vi "HeadAcousticHDF_Create.vi"(0 "reference in":refnum<class "HeadAcousticHDF.lvclass">, 5 "error in (no error)":errorcluster, 6 "Time Data":refnum<class "GSwFormDSP.lvclass">, 7 "Application Name":string, 9 "State Queue":string[](array[string])) -> (14 "reference out":refnum<class "HeadAcousticHDF.lvclass">, 19 "error out":errorcluster)   [LabVIEW 2022 SP3, in "HeadAcousticHDF.lvclass"]
doc: "Constructor."
uses:
  HeadAcousticHDF.lvclass
  C:/Program Files/National Instruments/LabVIEW 2022/vi.lib/addons/_AddQ/G#Object/G#Object.lvclass
  W:/projects/archives/23 Charette AI Group/SPWB/API/Generic Utilities_class/Generic Utilities.lvclass
  API/GSwFormDSP_class/GSwFormDSP.lvclass
  <vilib>/addons/_AddQ/G#Object/G#Object.lvclass
  API/Generic Utilities_class/Generic Utilities.lvclass
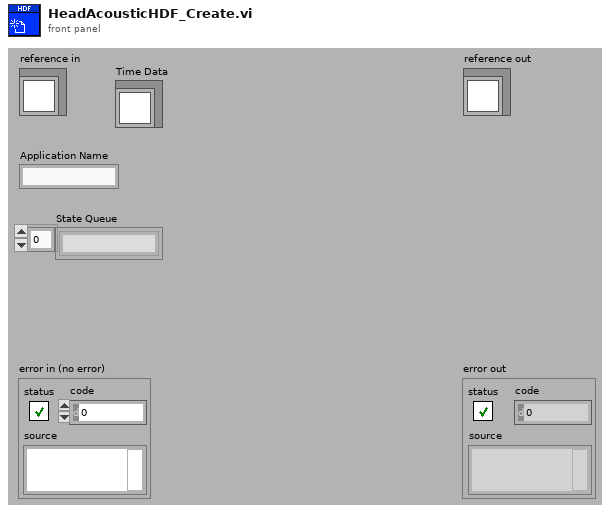
[diagram p1: front panel]
types:
  T1 = typedef "HeadAcousticHDF.lvclass/ObjectAttributesRef.ctl" = refnum<data-value>
  T2 = typedef "HeadAcousticHDF.lvclass/ObjectAttributes.ctl" = cluster{"Time Data":refnum<class "GSwFormDSP.lvclass">, "Data Plugin Name":string, "Additional Data Plugin Name":string, "New Time Data Obj?":bool}
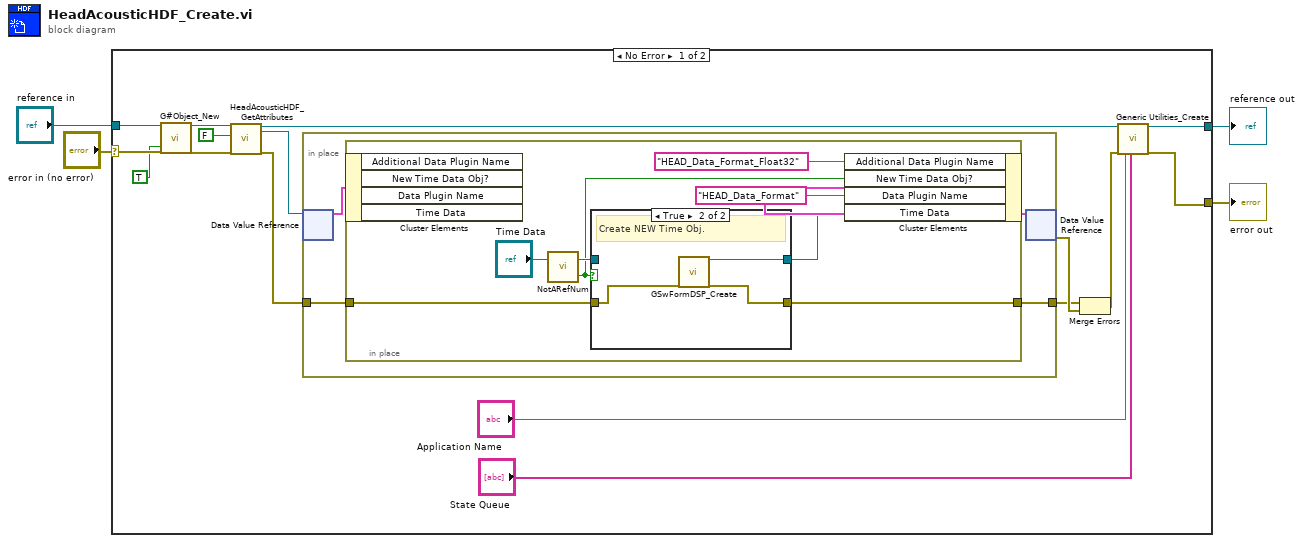
[diagram p0: block diagram]
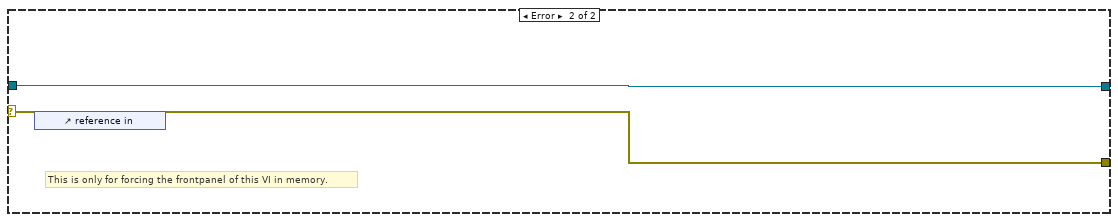
[diagram p3: hidden frame]
diagram:
  n1 = case shown="No Error" "error in (no error)" {
    selector: "error in (no error)" -> [w19 w39]
    tunnel: [w9 w39] -> w3
    tunnel: [w11 w38] -> w1
    tunnel: "reference in" -> [w20 w38]
    frame No Error {
      n2 = call <vilib>:"G#Object_New.vi"("reference in"=w20, "error in (no error)"=w19, "user counter (T)?"=TRUE ("User Counter")) -> ("reference out"=w14:refnum<class "HeadAcousticHDF.lvclass">, "error out"=w13:errorcluster)  [unwired: 14 in, 1 out]
      n3 = call "HeadAcousticHDF_GetAttributes.vi"("reference in"=w14, "return data? (T)"=FALSE ("return data"), "error in (no error)"=w13) -> ("reference out"=w12:refnum<class "HeadAcousticHDF.lvclass">, "attributes ref"=w16:T1, "error out"=w7:errorcluster)  [unwired: 13 in, 1 out]
      n4 = in-place {
        in-place-border: w7 -> [w22]
        in-place-border: [w21] -> w6
        n5 = in-place-dvr #1(w16) -> (w23:T2)  [unwired: 1 out]
        n6 = in-place {
          in-place-border: w22 -> [w30]
          in-place-border: [w29] -> w21
          n7 = in-place-cluster #2(w23) -> ()  [unwired: 4 out]
          n8 = call-dynamic "NotARefNum.vi"("reference in"="Time Data") -> ("not a refnum?"=w27:bool, "reference out"=w32:refnum<class "GSwFormDSP.lvclass">)  [unwired: 1 in]
          n9 = case shown="True" w27 {
            tunnel: [w34 w37] -> w25
            tunnel: w32 -> [w34 _]
            tunnel: w30 -> [w33 w36]
            tunnel: [w33 w35] -> w29
            frame False {
              # "Copy an existing reference."
            }
            frame True {
              # "Create NEW Time Obj."
              n10 = call "GSwFormDSP_Create.vi"("error in (no error)"=w36) -> ("reference out"=w37:refnum<class "GSwFormDSP.lvclass">, "error out"=w35:errorcluster)  [unwired: 17 in]
            }
          }
          n11 = in-place-cluster #2("Additional Data Plugin Name"="HEAD_Data_Format_Float32" ("Data Plugin Name"), "New Time Data Obj?"=w27, "Data Plugin Name"="HEAD_Data_Format", "Time Data"=w25) -> (w24:T2)
        }
        n12 = in-place-dvr #1(w24) -> (w17:errorcluster)  [unwired: 1 out]
      }
      n13 = Merge Errors(w6, w17) -> (w10:errorcluster)
      n14 = call "Generic Utilities_Create.vi"("reference in"=w12, "error in (no error)"=w10, "Application Name"="Application Name", "State Queue"="State Queue") -> ("reference out"=w11:refnum<class "HeadAcousticHDF.lvclass">, "error out"=w9:errorcluster)  [unwired: 14 in]
    }
    frame Error {
      # "This is only for forcing the frontpanel of this VI in memory."
      n15 = control-ref of="reference in"() -> ()  [unwired: 1 out]
    }
  }
  "error out" <- w3
  "reference out" <- w1
